vi "timing structure.vi"() -> ()   [LabVIEW 2018, in "Application.lvlib"]
uses:
  Application.lvlib
panel:
  in  "T2":dbl
  in  "T1":u32
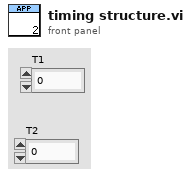
[diagram p1: front panel]
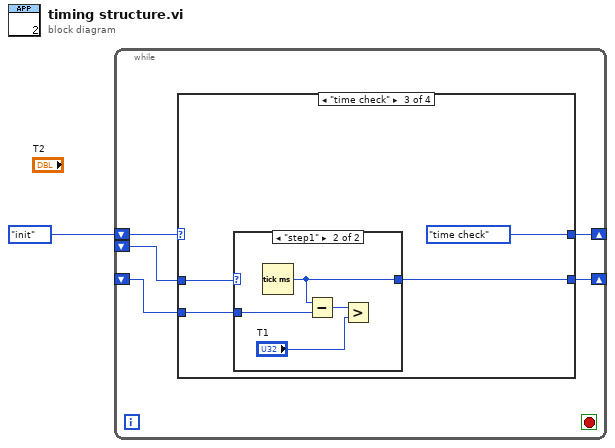
[diagram p0: block diagram]
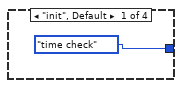
[diagram p2: hidden frame]
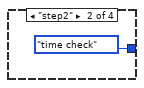
[diagram p3: hidden frame]
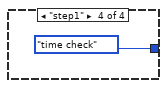
[diagram p5: hidden frame]
diagram:
  n1 = while {
    shift-right: [w5] -> _
    shift-left: enum16{"init", "step1", "step2", "time check"}."init" -> [w6]
    shift-left: _ -> [w4]
    shift-right: [w3] -> _
    shift-left: _ -> [w2]
    stop <- _ stop-if-true
    n2 = case shown="\"time check\"" w6 {
      tunnel: [enum16{"init", "step1", "step2", "time check"}."time check" enum16{"init", "step1", "step2", "time check"}."time check" enum16{"init", "step1", "step2", "time check"}."time check" enum16{"init", "step1", "step2", "time check"}."time check"] -> w5
      tunnel: w4 -> [_ _ w11 _]
      tunnel: [_ _ w10 _] -> w3
      tunnel: w2 -> [_ _ w9 _]
      frame "init", Default {
      }
      frame "step2" {
      }
      frame "time check" {
        n3 = case shown="\"step1\"" w11 {
          tunnel: [_ w16] -> w10
          tunnel: w9 -> [_ w15]
          frame "init", Default {
          }
          frame "step1" {
            n4 = Tick Count (ms)() -> (millisecond timer value=w16:u32)
            n5 = Subtract(x=w16, y=w15) -> (x-y=w13:u32)
            n6 = Greater?(x=w13, y="T1") -> ()  [unwired: 1 out]
          }
        }
      }
      frame "step1" {
      }
    }
  }
